vi "Weather_StatErr_Message.vi"(1 "Message number":i32 min=0 step=1) -> (0 "Status/Error string":string)   [LabVIEW 2013]
uses:
  Globals/Status_Error_Messages.vi
  Globals/Weather_Queues.vi
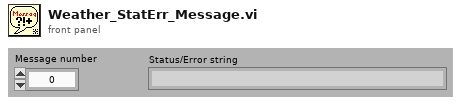
[diagram p1: front panel]
types:
  T1 = cluster{"Weather data (5s)":refnum<queue>, "Database queue":refnum<queue>, "Message queue":refnum<queue>, "Settings queue":refnum<queue>, "60 mins data queue":refnum<queue>, "48 hrs data queue":refnum<queue>}
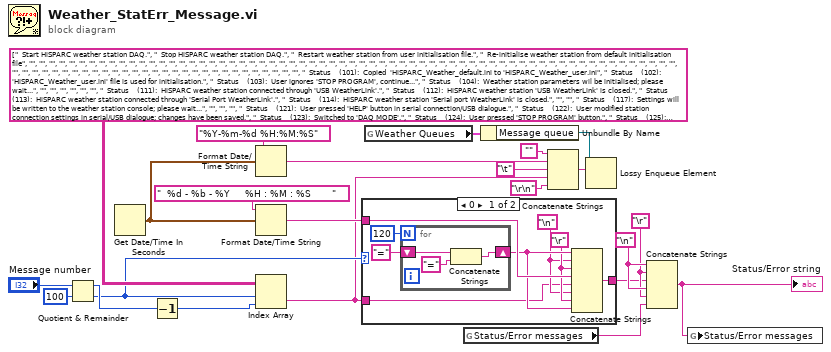
[diagram p0: block diagram]
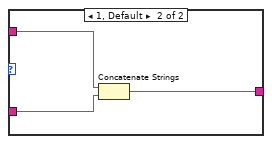
[diagram p2: hidden frame]
diagram:
  w21 = "\n"
  w20 = "\r"
  n1 = Quotient & Remainder(x="Message number", y=100) -> (x-y*floor(x/y)=w16:i32, floor(x/y)=w12:i32)
  n2 = Get Date/Time In Seconds() -> (seconds since 1Jan1904=w4:timestamp)
  n3 = Decrement(x=w16) -> (x-1=w13:i32)
  n4 = Format Date/Time String(time format string (%c)="%Y-%m-%d %H:%M:%S", seconds (now)=w4) -> (date/time string=w6:string)  [unwired: 1 out]
  n5 = Format Date/Time String(time format string (%c)="  %d - %b - %Y     %H : %M : %S       ", seconds (now)=w4) -> (date/time string=w22:string)  [unwired: 1 in]
  n6 = Index Array(array=string[][] [["  Start HiSPARC weather station DAQ.", "  Stop HiSPARC weather station DAQ.", "  Restart weather station from user initialisation file.", "  Re-initialise weather station from default initialisation file", "", "", "", "", "", "", "", "", "", "", "", "", "", "", "", "", "", "", "", "", "", "", "", "", "", "", "", "", "", "", "", "", "", "", "", "", "", "", "", "", "", "", "", "", "", "", "", "", "", "", "", "", "", "", "", "", "", "", "", "", "", "", "", "", "", "", "", "", "", "", "", "", "", "", "", "", "", "", "", "", "", "", "", "", "", "", "", "", "", "", "", "", "", ""], ["  Status    (101):  Copied  'HiSPARC_Weather_default.ini to 'HiSPARC_Weather_user.ini", "  Status    (102):  'HiSPARC_Weather_user.ini' file is used for initialisation.", "  Status    (103):  User ignores 'STOP PROGRAM', continue...", "  Status    (104):  Weather station parameters wil be initialised; please wait...", "", "", "", "", "", "", "  Status    (111):  HiSPARC weather station connected through 'USB WeatherLink'.", "  Status    (112):  HiSPARC weather station 'USB WeatherLink' is closed.", "  Status    (113):  HiSPARC weather station connected through 'Serial Port WeatherLink'.", "  Status    (114):  HiSPARC weather station 'Serial port WeatherLink' is closed.", "", "", "  Status    (117):  Settings will be written to the weather station console; please wait...", "", "", "", "  Status    (121):  User pressed 'HELP' button in serial connection/USB dialogue.", "  Status    (122):  User modified station connection settings in serial/USB dialogue; changes have been saved.", "  Status    (123):  Switched to 'DAQ MODE'.", "  Status    (124):  User pressed 'STOP PROGRAM' button.", "  Status    (125):  (New) settings have been saved.", "  Status    (126):  User pressed 'CALIBRATE' button; please wait until settings have been uploaded...", "  Status    (127):  User skips weather station calibration, continue...", "  Status    (128):  User pressed 'RESET' button but skips reset.", "  Status    (129):  User pressed 'HELP' button.", "  Status    (130):  Switched to 'STOP DAQ' mode.", "  Status    (131):  Weather station DAQ starts in 'DAQ MODE'.", "", "", "", "", "  Status    (136):  Calibration: latitude and/or longitude have not been modified.", "  Status    (137):  Calibration: temperature and/or humidity offset(s) have not been modified.", "  Status    (138):  Calibration: sea level barometer and/or station elevation have not been modified.", "  Status    (139):  Calibration: wind direction offset has not been modified.", "", "  Status    (141):  Weather station console successfully initialised.", "", "", "", "", "", "", "", "", "  Status    (150):  Weather sensor units are correctly set; no modifications required.", "", "", "", "", "  Status    (155):  Rain collector model correctly set ('0.2 mm'); no modification required.", "", "", "", "", "", "", "", "", "", "  Status    (165):  Wind cup size correctly set ('large'); no modification required.", "", "", "", "", "  Status    (170):  Time on weather station console correctly set (= pc time); no modification required.", "", "", "", "", "  Status    (175):  Calibration: station latititude and longitude match console settings; no adjustment required.", "", "", "", "", "  Status    (180):  Calibration: wind direction offset matches console settings; no adjustment required.", "", "", "", "", "  Status    (185):  Calibration: temperature and humidity offset(s) match console settings; no adjustment required.", "", "", "", "", "", "", "", "", "", "", "", "", ""], ["  Warning (201):  No GPS time correction in HiSPARC.ini (correction = 0 s)!", "  Warning (202):  PC clock time error in HiSPARC.ini (GPS time correction is set to 0 s)!", "  Warning (203):  Error in GPS time stamp in HiSPARC.ini (GPS time correction is set to 0 s)!", "  Warning (204):  Unknown message in HiSPARC.ini (GPS time correction is set to 0 s)!", "  Warning (205):  Time difference too large in HiSPARC.ini (GPS time correction is set to 0 s)!", "", "", "", "", "", "  Warning (211):  Cannot open HiSPARC weather station connection through 'USB WeatherLink'!", "  Warning (212):  Cannot close HiSPARC weather station connection through 'USB WeatherLink'!", "  Warning (213):  Cannot open HiSPARC weather station connection through 'Serial Port WeatherLink'!", "  Warning (214):  Cannot close HiSPARC weather station connection through 'Serial Port WeatherLink'!", "  Warning (215):  Station ID = 0; please select a valid station number!", "  Warning (216):  No USB connection or Serial COM port number = 0; please check or select a valid port number!", "  Warning (217):  Try automatic reconnection to HiSPARC weather station console!", "", "", "", "  Warning (221):  Please check your internet connection; cannot reach HiSPARC document server!", "  Warning (222):  User pressed 'STOP PROGRAM' button in serial/USB dialogue!", "  Warning (223):  Overflow event queue for buffer database; 1 event is lost!", "  Warning (224):  Overflow event queue for front panel graphs!", "", "  Warning (226):  No modification(s); proposed calibration parameters equal calibration parameters on console!", "", "  Warning (228):  User pressed 'RESET' button; restart with default settings!", "", "", "  Warning (231):  Failed to set timeout/read weather station and/or DLL/Firmware version/date, will retry!", "  Warning (232):  Failed to initialise weather sensor units, will retry!", "  Warning (233):  Failed to set rain collector model to '0.2 mm', will retry!", "  Warning (234):  Failed to set wind cup size to 'large', will retry!", "  Warning (235):  Failed to synchronise pc clock and weather station clock, will retry!", "  Warning (236):  Calibration: failed to set latitude and/or longitude, will retry!", "  Warning (237):  Calibration: failed to set temperature and/or humidity offset(s), will retry!", "  Warning (238):  Calibration: failed to set sea level barometer and/or station elevation, will retry!", "  Warning (239):  Calibration: failed to set wind direction offset, will retry!", "", "  Warning (241):  Failed to initialise weather station console, will retry!", "", "", "", "", "", "", "", "", "  Warning (250):  Weather sensor units have successfully been modified!", "", "", "", "", "  Warning (255):  Rain collector model has successfully been set to '0.2 mm'!", "", "", "", "", "", "", "", "", "", "  Warning (265):  Wind cup size has successfully been set to 'large'!", "", "", "", "", "  Warning (270):  Time on weather station console has successfully been set to pc time!", "", "", "", "", "  Warning (275):  Calibration: station latititude and/or longitude have successfully been modified!", "", "", "", "", "  Warning (280):  Calibration: wind direction offset has successfully been modified!", "", "", "", "", "  Warning (285):  Calibration: temperature and/or humidity offset(s) have successfully been modified!", "", "", "", "", "", "", "  Warning (292):  Calibration: sea level barometer value and station elevation have successfully been reset to factory settings!", "", "", "  Warning (295):  Calibration: sea level barometer value has successfully been modified!", "", "", "  Warning (298):  Calibration: station elevation has successfully been modified!"], ["  Error      (301):  Path to HiSPARC weather station DAQ software has not been found!", "  Error      (302):  Initialisation file 'HiSPARC.ini' has not been found!", "  Error      (303):  Initialisation file 'HiSPARC_Weather_default.ini' has not been found!", "  Error      (304):  Failed copying  'HiSPARC_Weather_default.ini' to 'HiSPARC_Weather_user.ini'!", "", "  Error      (306):  Error in reading parameters from HiSPARC.ini!", "", "", "", "", "", "", "", "", "", "", "", "", "", "", "", "  Error      (322):  Lost connection to weather station; will automatically try to reconnect!", "  Error      (323):  Cannot connect to buffer database!", "", "", "", "", "", "", "  Error      (330):  Failed to initialise weather station supporting software library (DLL), quit!", "", "", "", "", "", "", "", "", "", "  Error      (340):  This weather station model is not supported!", "  Error      (341):  Failed to initialise weather station console several times, quit!", "", "", "", "", "", "", "", "", "  Error      (350):  Failed to read weather sensor units!", "  Error      (351):  Failed to write weather sensor units!", "  Error      (352):  Failed to read weather sensor units after modification!", "  Error      (353):  Failed to match weather sensor units after write/read operation!", "", "  Error      (355):  Failed to read rain collector model!", "  Error      (356):  Failed to write rain collector model!", "  Error      (357):  Failed to read rain collector model after modification!", "  Error      (358):  Failed to match rain collector model after write/read operation!", "  Error      (359):  Failed to set rain collector model ('0.2 mm') on console!", "  Error      (360):  Failed to read rain collector model from console after modification!", "  Error      (361):  Failed to match rain collector model from console after modification!", "  Error      (362):  Failed to read rain collector model from console!", "", "", "  Error      (365):  Failed to read wind cup size!", "  Error      (366):  Failed to write wind cup size!", "  Error      (367):  Failed to read wind cup size after modification!", "  Error      (368):  Failed to set wind cup size to 'large'; please check/modify cup size on the weather station console!", "", "  Error      (370):  Failed to read time from weather station console!", "  Error      (371):  Failed to write pc time to weather station console!", "  Error      (372):  Failed to read time from weather station console after modification!", "  Error      (373):  Failed to match time from weather station console after write/read operation!", "", "  Error      (375):  Calibration: failed to read station latitude and/or longitude!", "  Error      (376):  Calibration: failed to write station latitude!", "  Error      (377):  Calibration: failed to write station longitude!", "  Error      (378):  Calibration: failed to read station latitude and/or longitude after modification!", "  Error      (379):  Calibration: failed to match station latitude and/or longitude after write/read operation!", "  Error      (380):  Calibration: failed to read wind direction offset!", "  Error      (381):  Calibration: failed to write wind direction offset!", "  Error      (382):  Calibration: failed to read wind direction offset after modification!", "  Error      (383):  Calibration: failed to match wind direction offset after write/read operation!", "", "  Error      (385):  Calibration: temperature and/or humidity offset(s) out of range!", "  Error      (386):  Calibration: failed to load temperature and/or humidity calibration data from console!", "  Error      (387):  Calibration: failed to write temperature and/or humidity offset(s) after modification!", "  Error      (388):  Calibration: failed to store temperature and/or humidity offset(s) into console!", "  Error      (389):  Calibration: failed to match temperature and/or humidity offset(s) after write/read operation!", "  Error      (390):  Calibration: failed to write sea level barometer value and/or station elevation!", "  Error      (391):  Calibration: failed to read sea level barometer value and/or station elevation!", "  Error      (392):  Failed to set sea level barometer and station elevation; please check/modify them on the weather station console!", "  Error      (393):  Calibration: failed to write sea level barometer value!", "  Error      (394):  Calibration: failed to read sea level barometer value after modification!", "  Error      (395):  Calibration: failed to match sea level barometer value after write/read operation!", "  Error      (396):  Calibration: failed to write station elevation!", "  Error      (397):  Calibration: failed to read station elevation after modification!", "  Error      (398):  Calibration: failed to match station elevation after write/read operation!"]], index (row)=w12, index (col)=w13) -> (element=w2:string)
  n7 = case shown="0" w12 {
    tunnel: w22 -> [w30 w37]
    tunnel: w2 -> [w25 w36]
    tunnel: [w29 w35] -> w11
    frame 0 {
      w26 = "\n"
      w27 = "\r"
      n8 = for {
        N: 120 -> [_]
        shift-right: [w32] -> w28
        shift-left: "=" -> [w34]
        n9 = Concatenate Strings(w34, "=" ("string")) -> (w32:string)
      }
      n10 = Concatenate Strings(w28, w26, w27, w30, w25, w26, w27, w28) -> (w29:string)
    }
    frame 1, Default {
      n11 = Concatenate Strings(w37, w36) -> (w35:string)
    }
  }
  n12 = global read "Weather_Queues.vi" "Weather Queues"() -> (w10:T1)
  n13 = global read "Status_Error_Messages.vi" "Status/Error messages"() -> (w15:string)
  n14 = Unbundle By Name(w10) -> ("Message queue"=w9:refnum<queue>)
  n15 = Concatenate Strings("", w6, "\t", w2, "\r\n") -> (w5:string)
  n16 = Lossy Enqueue Element(queue=w9, element=w5) -> ()  [unwired: 1 in, 4 out]
  n17 = Concatenate Strings(w21, w20, w11, w21, w20, w15) -> (w14:string)
  "Status/Error string" <- w14
  n18 = global write "Status_Error_Messages.vi" "Status/Error messages"(w14) -> ()
